vi "DigitalInOut_read.vi"(8 "error in (no error)":errorcluster, 11 "DigitalInOut in":refnum<class "DigitalInOut.lvclass">) -> (0 "error out":errorcluster, 2 "value":bool, 3 "DigitalInOut out":refnum<class "DigitalInOut.lvclass">)   [LabVIEW 2011, in "mbed_LVLibrary.lvlib" / "DigitalInOut.lvclass"]
uses:
  DigitalInOut.lvclass
  DigitalInOut.lvclass/DigitalInOut.ctl
  Transport Mechanisms/mbed/mbed.lvclass
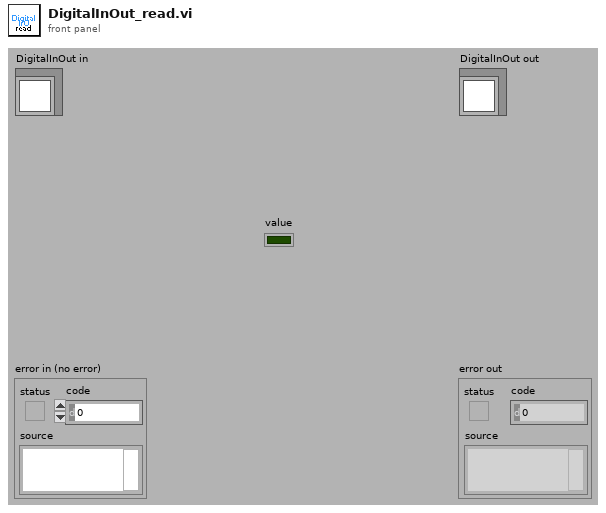
[diagram p1: front panel]
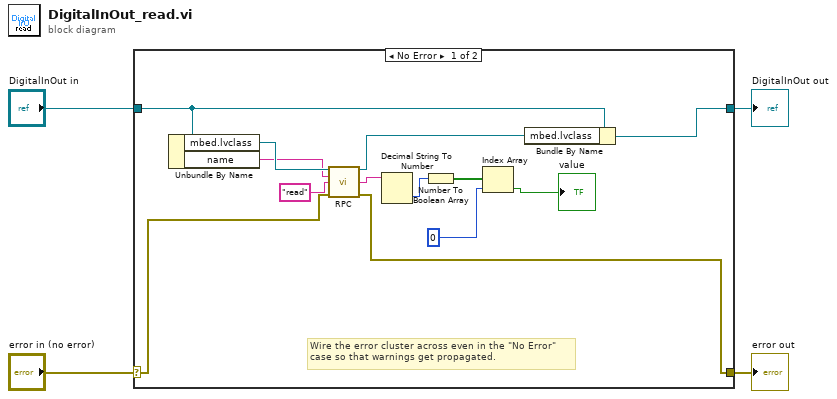
[diagram p0: block diagram]
diagram:
  n1 = case shown="No Error" "error in (no error)" {
    selector: "error in (no error)" -> [w6 w19]
    tunnel: [w5 w19] -> w3
    tunnel: [w8 w18] -> w1
    tunnel: "DigitalInOut in" -> [w9 w18]
    frame No Error {
      # "Wire the error cluster across even in the \"No Error\"\ncase so that warnings get propagated."
      n2 = Unbundle By Name(w9) -> ("mbed.lvclass"=w13:refnum<class "mbed.lvclass">, "name"=w12:string)
      n3 = call-dynamic "RPC.vi"("mbed in"=w13, "Name"=w12, "method"="read", "error in (no error)"=w6) -> ("mbed out"=w7:refnum<class "mbed.lvclass">, "RPC Result"=w16:string, "error out"=w5:errorcluster)  [unwired: 9 in]
      n4 = Decimal String To Number(string=w16) -> (number=w14:i32)  [unwired: 2 in, 1 out]
      n5 = Number To Boolean Array(number=w14) -> (Boolean array=w11:bool[])
      n6 = Index Array(array=w11, index=0) -> (element=→"value":bool)
      n7 = Bundle By Name(cluster=w9, "mbed.lvclass"=w7) -> (w8:refnum<class "DigitalInOut.lvclass">)
    }
    frame Error {
    }
  }
  "error out" <- w3
  "DigitalInOut out" <- w1
